vi "Build Module.vi"() -> ()   [LabVIEW 2016]
uses:
  Classes/Assembly/Assembly Run.lvclass
  Classes/Routine/Routine Enum.ctl
  Classes/Routine/Routine.lvclass
  Classes/Workspace/Fixture Enum.ctl
  Classes/Workspace/Fixture.lvclass
  Classes/Controller/Controller.lvclass
  Status.vi
panel:
  out "Routines":string[](array[string])
  out "Status":T1
  in  "Open I/O Test":bool
  in  "Run":bool
  in  "Glue step":enum16{"Kapton", "Sensor", "PCB"}(ring)
  in  "Add":bool
  in  "Number of modules":i32
  in  "Component Tray ID":i32
  in  "Baseplate Tray ID":i32
  in  "Stop":bool
  # "Vacuum Test"
  # "Assembly Controls"
  # "Region 3"
  # "Region 2"
  # "Region 1"
  # "Position 2"
  # "Position 1"
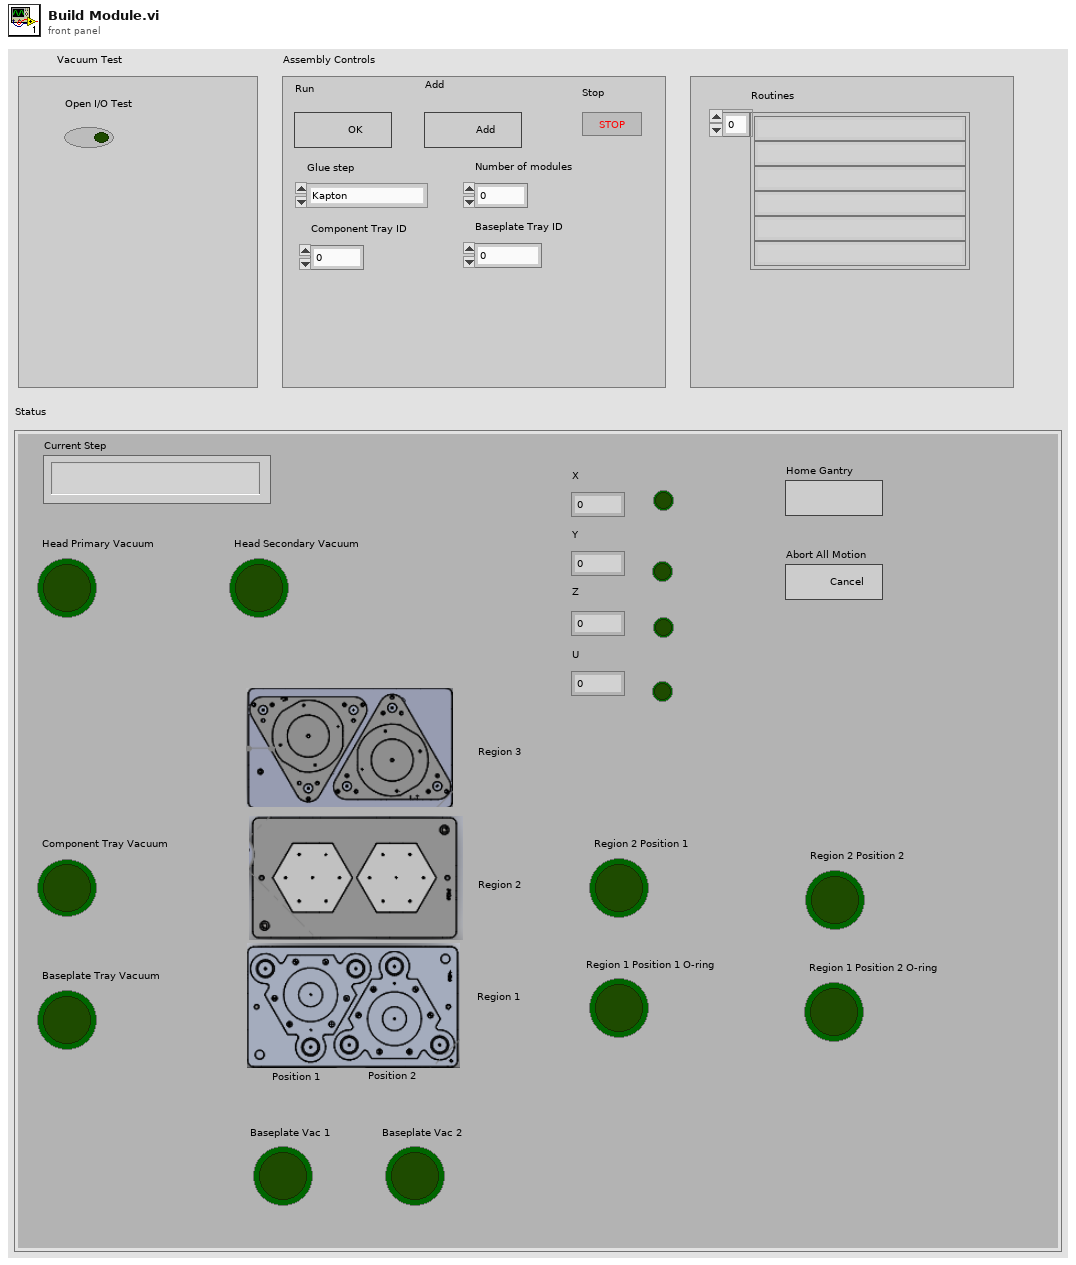
[diagram p1: front panel]
types:
  T1 = cluster{"Current Step":string, "Baseplate Tray Vacuum":bool, "Component Tray Vacuum":bool, "Head Primary Vacuum":bool, "Head Secondary Vacuum":bool, "Region 1 Position 1 O-ring":bool, "Region 1 Position 2 O-ring":bool, "Region 2 Position 1":bool, "Region 2 Position 2":bool, "X":dbl, "Y":dbl, "Z":dbl, "U":dbl, "Home Gantry":bool, bool, bool, bool, bool, "Abort All Motion":bool, "Baseplate Vac 1":bool, "Baseplate Vac 2":bool}
  T2 = cluster{"Current Step":string, "Baseplate Tray Vacuum":bool, "Component Tray Vacuum":bool, "Head Primary Vacuum":bool, "Head Secondary Vacuum":bool, "Region 1 Position 1 O-ring":bool, "Region 1 Position 2 O-ring":bool, "Region 2 Position 1":bool, "Region 2 Position 2":bool, "X":dbl, "Y":dbl, "Z":dbl, "U":dbl, "Home Position":bool, "Enabled":bool, "Enabled 2":bool, bool, bool, "Abort All Motion":bool, "Baseplate Vac 1":bool, "Baseplate Vac 2":bool}
  T3 = enum32{"Invalid", "Standard", "Closed", "Hidden", "Minimized", "Maximized"}
  T4 = typedef "Fixture.lvclass/Fixture Enum.ctl" = enum16{"Assembly Tray", "Syringe Space", "Component", "Pick Up Tool", "Current Position"}
  T5 = typedef "Routine.lvclass/Routine Enum.ctl" = enum16{"Primary Pick Up", "Pick Up All", "Put Down Secondary", "Put Down All", "Release Syringe", "Secondary Pick Up", "Secure Syringe", "Dispense on Plate", "Dispense on Kapton", "Dispense on Sensor"}
  T6 = typedef "Controller.lvclass/Controllers.ctl" = cluster{"I-O.lvclass":refnum<class "I-O.lvclass">, "Motion.lvclass":refnum<class "Motion.lvclass">, "Dispenser.lvclass":refnum<class "Dispenser.lvclass">}
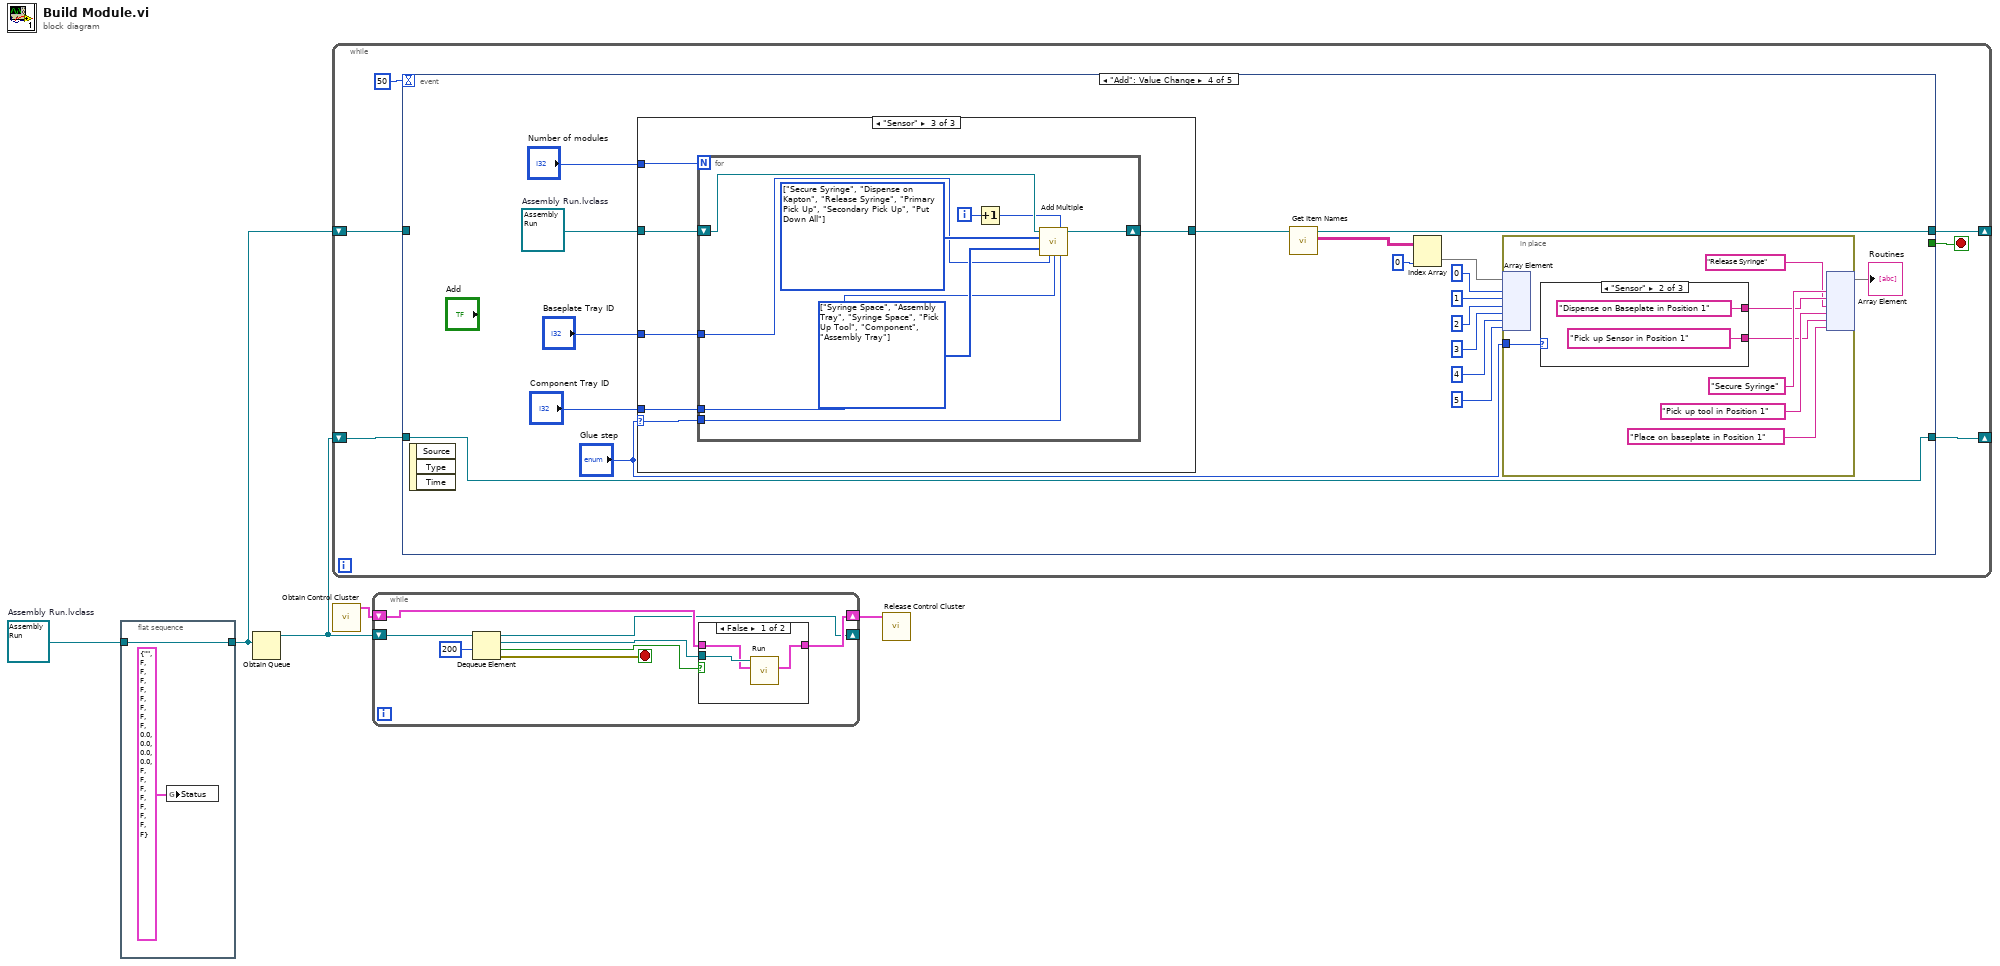
[diagram p0: block diagram]
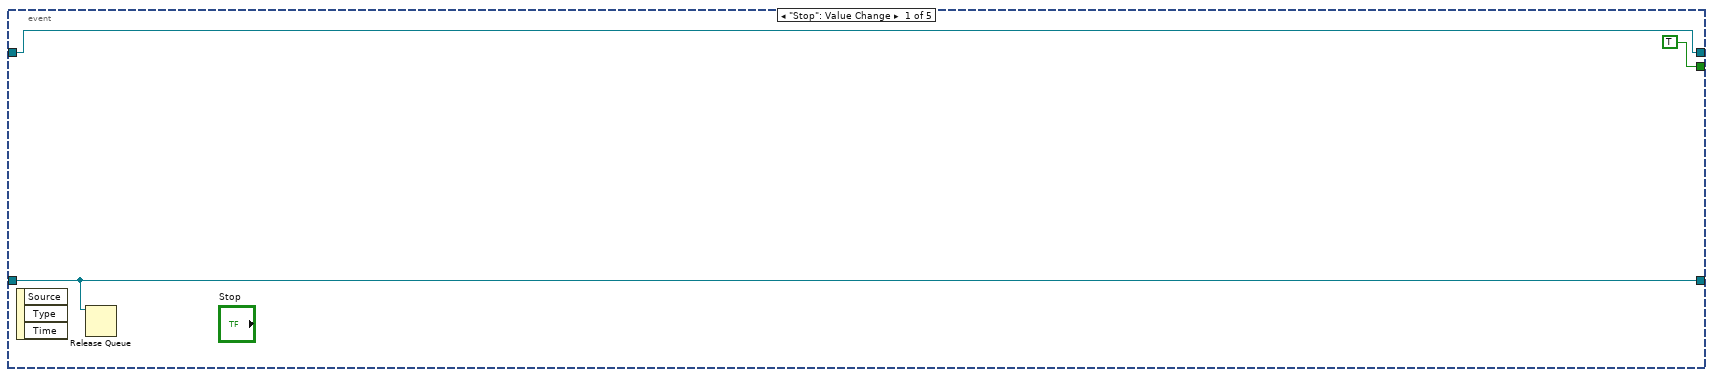
[diagram p3: hidden frame]
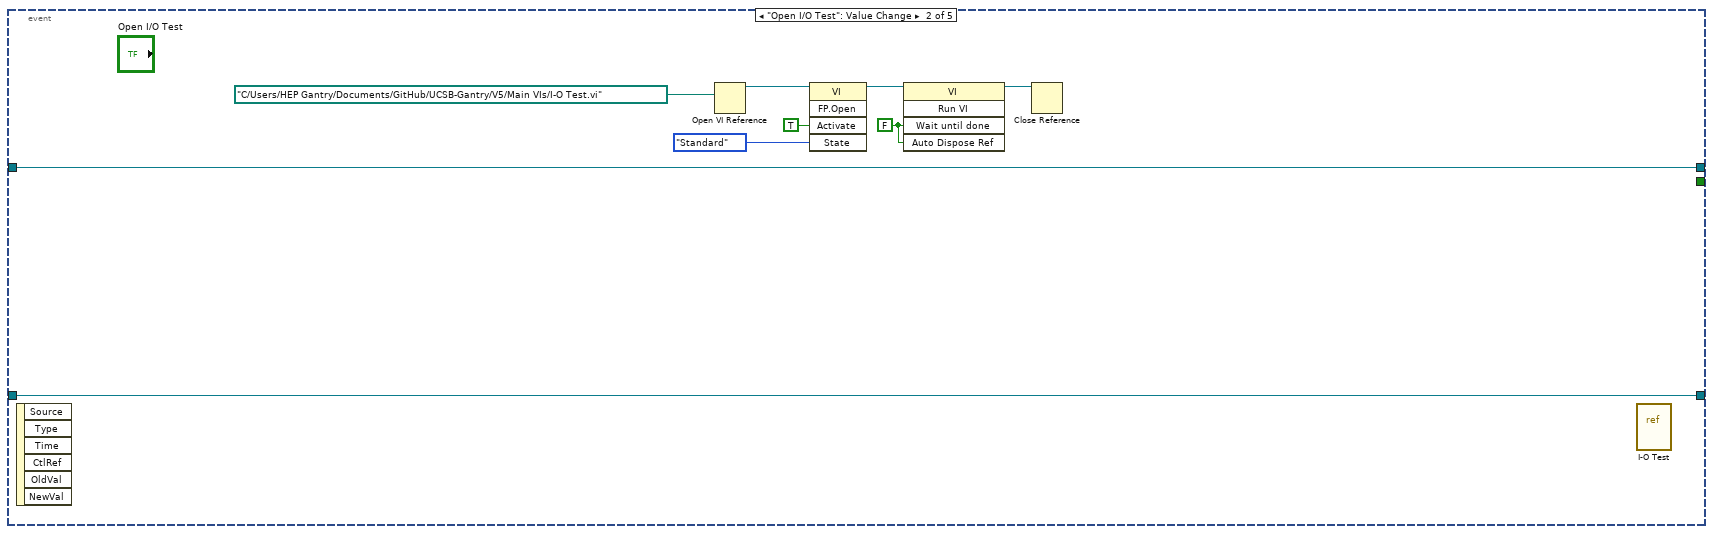
[diagram p4: hidden frame]
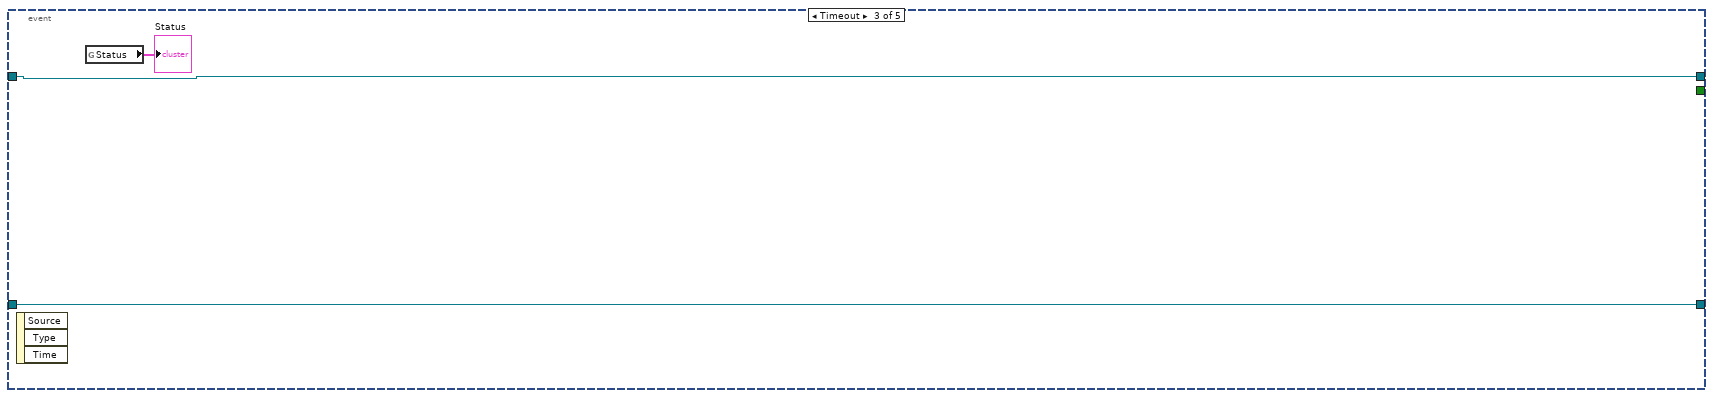
[diagram p5: hidden frame]
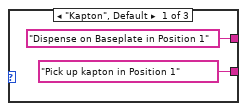
[diagram p6: hidden frame]
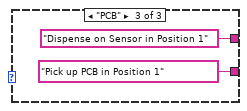
[diagram p7: hidden frame]
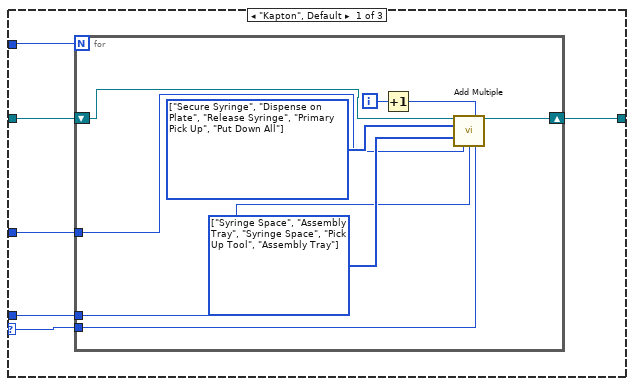
[diagram p8: hidden frame]
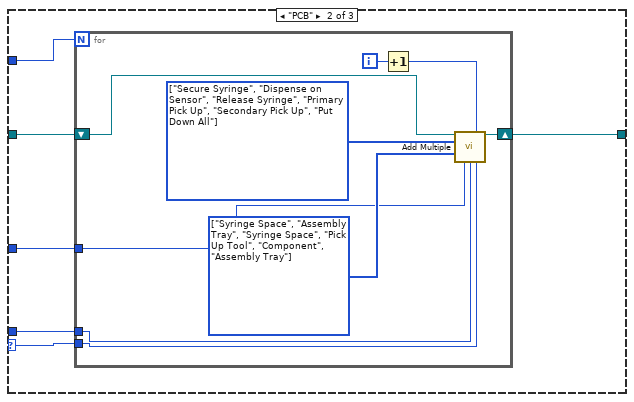
[diagram p9: hidden frame]
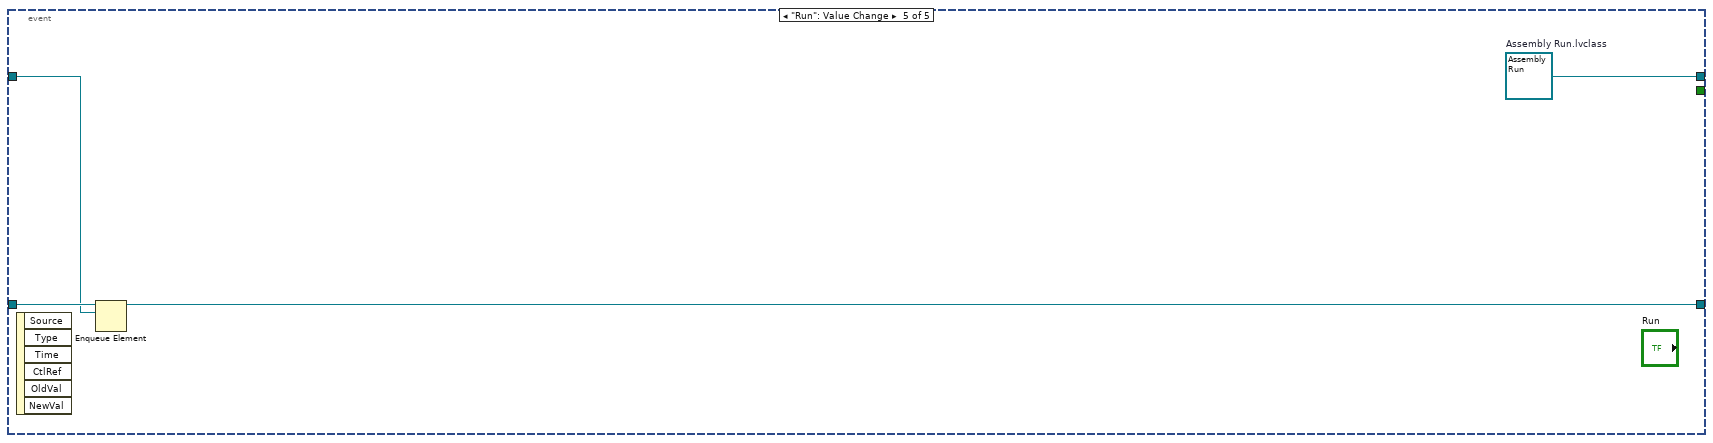
[diagram p10: hidden frame]
diagram:
  w2 = refnum<class "Assembly Run.lvclass"> refnum  # Assembly Run.lvclass
  n1 = flat-sequence {
    tunnel: w2 -> [w6]
    tunnel: [w6] -> w1
    frame #0 {
      n2 = global write "Status.vi" "Status"(T2 {"Current Step"="", "Baseplate Tray Vacuum"=FALSE, "Component Tray Vacuum"=FALSE, "Head Primary Vacuum"=FALSE, "Head Secondary Vacuum"=FALSE, "Region 1 Position 1 O-ring"=FALSE, "Region 1 Position 2 O-ring"=FALSE, "Region 2 Position 1"=FALSE, "Region 2 Position 2"=FALSE, "X"=0.0, "Y"=0.0, "Z"=0.0, "U"=0.0, "Home Position"=FALSE, "Enabled"=FALSE, "Enabled 2"=FALSE, FALSE, FALSE, "Abort All Motion"=FALSE, "Baseplate Vac 1"=FALSE, "Baseplate Vac 2"=FALSE} ("Status")) -> ()
    }
  }
  n3 = Obtain Queue(element data type=w1) -> (queue out=w5:refnum<queue>)  [unwired: 4 in, 2 out]
  n4 = while {
    shift-right: [w12] -> _
    shift-left: w5 -> [w13]
    shift-right: [w10] -> _
    shift-left: w1 -> [w9]
    stop <- w11 stop-if-true
    n5 = event shown="[3] \"Add\": Value Change" {
      selector: _ -> [_ _ _ _ _]
      dyn-events: _ -> [_ _ _ _ _]
      timeout: 50 -> [_ _ _ _ _]
      tunnel: w13 -> [w14 w23 w27 w45 w107]
      tunnel: [w14 w23 w27 w45 w105] -> w12
      tunnel: [TRUE _ _ _ _] -> w11
      tunnel: [w15 w24 w28 w40 w108] -> w10
      tunnel: w9 -> [w15 w24 w28 _ w106]
      event "Stop": Value Change {
        n6 = event-data() -> ()  [unwired: 1 in, 3 out]
        n7 = Release Queue(queue=w14) -> ()  [unwired: 2 in, 3 out]
      }
      event "Open I/O Test": Value Change {
        w18 = FALSE
        n8 = event-data() -> ()  [unwired: 1 in, 6 out]
        n9 = Open VI Reference(vi path=path "C:/Users/HEP Gantry/Documents/GitHub/UCSB-Gantry/V5/Main VIs/I-O Test.vi") -> (vi reference=w22:refnum<vi>)  [unwired: 5 in, 1 out]
        n10 = invoke class="VI" method="FP.Open"(reference=w22, "Activate"=TRUE, "State"=T3."Standard") -> (reference out=w19:refnum<vi>)  [unwired: 2 in, 4 out]
        n11 = invoke class="VI" method="Run VI"(reference=w19, "Wait until done"=w18, "Auto Dispose Ref"=w18) -> (reference out=w17:refnum<vi>)  [unwired: 2 in, 4 out]
        n12 = Close Reference(reference=w17) -> ()  [unwired: 1 in, 1 out]
        n13 = vi-ref "I-O Test.vi"() -> ()  [unwired: 1 out]
      }
      event Timeout {
        n14 = event-data() -> ()  [unwired: 1 in, 3 out]
        n15 = global read "Status.vi" "Status"() -> (→"Status":T2)
      }
      event "Add": Value Change {
        w46 = refnum<class "Assembly Run.lvclass"> refnum  # Assembly Run.lvclass
        n16 = event-data() -> ()  [unwired: 1 in, 3 out]
        n17 = case shown="\"Sensor\"" "Glue step" {
          selector: "Glue step" -> [w60 w77 w90]
          tunnel: w46 -> [w64 w80 w91]
          tunnel: [w65 w79 w95] -> w41
          tunnel: "Number of modules" -> [w63 w78 w94]
          tunnel: "Component Tray ID" -> [w61 w76 w93]
          tunnel: "Baseplate Tray ID" -> [w62 w75 w92]
          frame "Kapton", Default {
            n18 = for {
              N: w63 -> [_]
              shift-right: [w73] -> w65
              shift-left: w64 -> [w74]
              tunnel: w62 -> [w68]
              tunnel: w61 -> [w67]
              tunnel: w60 -> [w66]
              i -> [w70]
              w72 = T4[] [enum."Syringe Space", enum."Assembly Tray", enum."Syringe Space", enum."Pick Up Tool", enum."Assembly Tray"] items=["Assembly Tray", "Syringe Space", "Component", "Pick Up Tool", "Current Position"] ("Fixtures")
              w71 = T5[] [enum."Secure Syringe", enum."Dispense on Plate", enum."Release Syringe", enum."Primary Pick Up", enum."Put Down All"] items=["Primary Pick Up", "Pick Up All", "Put Down Secondary", "Put Down All", "Release Syringe", "Secondary Pick Up", "Secure Syringe", "Dispense on Plate", "Dispense on Kapton", "Dispense on Sensor"] ("Routine")
              n19 = Increment(x=w70) -> (x+1=w69:i32)
              n20 = call-dynamic "Add Multiple.vi"("Assembly in"=w74, "Position"=w69, 5:w71, 9:w72, "Baseplate Tray ID"=w68, "Component Tray ID"=w67, "Glue step"=w66) -> ("Assembly out"=w73:refnum<class "Assembly Run.lvclass">)  [unwired: 7 in, 1 out]
            }
          }
          frame "PCB" {
            n21 = for {
              N: w78 -> [_]
              shift-right: [w88] -> w79
              shift-left: w80 -> [w89]
              tunnel: w77 -> [w85]
              tunnel: w76 -> [w84]
              tunnel: w75 -> [w83]
              i -> [w82]
              w86 = T4[] [enum."Syringe Space", enum."Assembly Tray", enum."Syringe Space", enum."Pick Up Tool", enum."Component", enum."Assembly Tray"] items=["Assembly Tray", "Syringe Space", "Component", "Pick Up Tool", "Current Position"] ("Fixtures")
              w87 = T5[] [enum."Secure Syringe", enum."Dispense on Sensor", enum."Release Syringe", enum."Primary Pick Up", enum."Secondary Pick Up", enum."Put Down All"] items=["Primary Pick Up", "Pick Up All", "Put Down Secondary", "Put Down All", "Release Syringe", "Secondary Pick Up", "Secure Syringe", "Dispense on Plate", "Dispense on Kapton", "Dispense on Sensor"] ("Routine")
              n22 = Increment(x=w82) -> (x+1=w81:i32)
              n23 = call-dynamic "Add Multiple.vi"("Assembly in"=w89, "Position"=w81, 5:w87, 9:w86, "Baseplate Tray ID"=w83, "Component Tray ID"=w84, "Glue step"=w85) -> ("Assembly out"=w88:refnum<class "Assembly Run.lvclass">)  [unwired: 7 in, 1 out]
            }
          }
          frame "Sensor" {
            n24 = for {
              N: w94 -> [_]
              shift-right: [w103] -> w95
              shift-left: w91 -> [w104]
              tunnel: w93 -> [w99]
              tunnel: w92 -> [w100]
              tunnel: w90 -> [w96]
              i -> [w98]
              w101 = T4[] [enum."Syringe Space", enum."Assembly Tray", enum."Syringe Space", enum."Pick Up Tool", enum."Component", enum."Assembly Tray"] items=["Assembly Tray", "Syringe Space", "Component", "Pick Up Tool", "Current Position"] ("Fixtures")
              w102 = T5[] [enum."Secure Syringe", enum."Dispense on Kapton", enum."Release Syringe", enum."Primary Pick Up", enum."Secondary Pick Up", enum."Put Down All"] items=["Primary Pick Up", "Pick Up All", "Put Down Secondary", "Put Down All", "Release Syringe", "Secondary Pick Up", "Secure Syringe", "Dispense on Plate", "Dispense on Kapton", "Dispense on Sensor"] ("Routine")
              n25 = Increment(x=w98) -> (x+1=w97:i32)
              n26 = call-dynamic "Add Multiple.vi"("Assembly in"=w104, "Position"=w97, 5:w102, 9:w101, "Baseplate Tray ID"=w100, "Component Tray ID"=w99, "Glue step"=w96) -> ("Assembly out"=w103:refnum<class "Assembly Run.lvclass">)  [unwired: 7 in, 1 out]
            }
          }
        }
        n27 = call "Get Item Names.vi"("Assembly Run in"=w41) -> ("Item names"=w39:string[][], "Assembly Run out"=w40:refnum<class "Assembly Run.lvclass">)  [unwired: 8 in, 1 out]
        n28 = Index Array(array=w39, index (col)=0 ("disabled index (col)")) -> (element=w37:string[])  [unwired: 1 in]
        n29 = in-place {
          in-place-border: "Glue step" -> [w48]
          n30 = in-place-array #1(w37, 0, 1, 2, 3, 4, 5) -> ()  [unwired: 6 out]
          n31 = case shown="\"Sensor\"" w48 {
            tunnel: ["Dispense on Baseplate in Position 1" "Dispense on Baseplate in Position 1" "Dispense on Sensor in Position 1"] -> w52
            tunnel: ["Pick up kapton in Position 1" "Pick up Sensor in Position 1" "Pick up PCB in Position 1"] -> w47
            frame "Kapton", Default {
            }
            frame "Sensor" {
            }
            frame "PCB" {
            }
          }
          n32 = in-place-array #1("Secure Syringe", w52, "Release Syringe", "Pick up tool in Position 1", w47, "Place on baseplate in Position 1") -> (→"Routines":string[])  [unwired: 6 out]
        }
      }
      event "Run": Value Change {
        w108 = refnum<class "Assembly Run.lvclass"> refnum  # Assembly Run.lvclass
        n33 = event-data() -> ()  [unwired: 1 in, 6 out]
        n34 = Enqueue Element(queue=w107, element=w106) -> (queue out=w105:refnum<queue>)  [unwired: 2 in, 2 out]
      }
    }
  }
  n35 = call "Obtain Control Cluster.vi"() -> ("Control Out"=w3:T6)  [unwired: 11 in]
  n36 = while {
    shift-right: [w109] -> _
    shift-left: w5 -> [w116]
    shift-right: [w111] -> w4
    shift-left: w3 -> [w112]
    stop <- w110 stop-if-true
    n37 = Dequeue Element(queue=w116, timeout in ms (-1)=200) -> (queue out=w109:refnum<queue>, element=w115:refnum<class "Assembly Run.lvclass">, timed out?=w114:bool, error out=w110:errorcluster)  [unwired: 1 in]
    n38 = case shown="False" w114 {
      tunnel: w115 -> [w119 _]
      tunnel: w112 -> [w118 w120]
      tunnel: [w117 w120] -> w111
      frame False {
        n39 = call-dynamic "Run.vi"("Control In"=w118, "Assembly In"=w119) -> ("Control Out"=w117:T6)  [unwired: 7 in, 2 out]
      }
      frame True {
      }
    }
  }
  n40 = call "Release Control Cluster.vi"("output cluster"=w4) -> ()  [unwired: 11 in]
